vi "control tab sliding.vi"(10 "close(T)/open(F)":bool, 11 "String":string) -> ()   [LabVIEW 2017]
doc: "SciScan 1.2 160622"
uses:
  GFG/GFGfpRefGet.vi
  GFG/GFGnumericGet.vi
  GFG/GFG library.lvlib
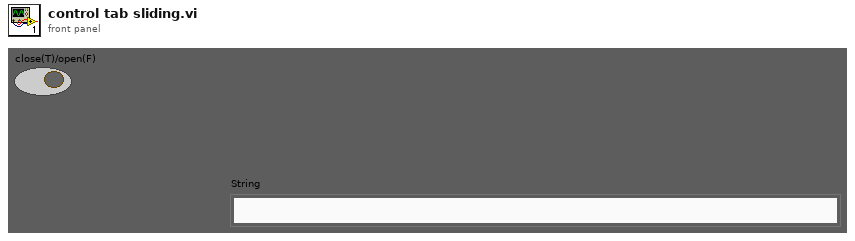
[diagram p1: front panel]
types:
  T1 = cluster{"WaveformChartRef":refnum<vi>, "DigitalRef":refnum<vi>, "ArrayRef":refnum<vi>, "TabControlRef":refnum<vi>, "EnumRef":refnum<vi>, "RingRef":refnum<vi>, "BooleanRef":refnum<vi>, "KnobRef":refnum<vi>, "SlideRef":refnum<vi>, "PathRef":refnum<vi>, "StringRef":refnum<vi>, "ComboBox":refnum<vi>, "WaveformGraphRef":refnum<vi>}
  T2 = cluster{"[0]":dbl, "[1]":dbl, "[2]":dbl, "[3]":dbl, "[4]":dbl, "[5]":dbl, "[6]":dbl, "[7]":dbl, "[8]":dbl}
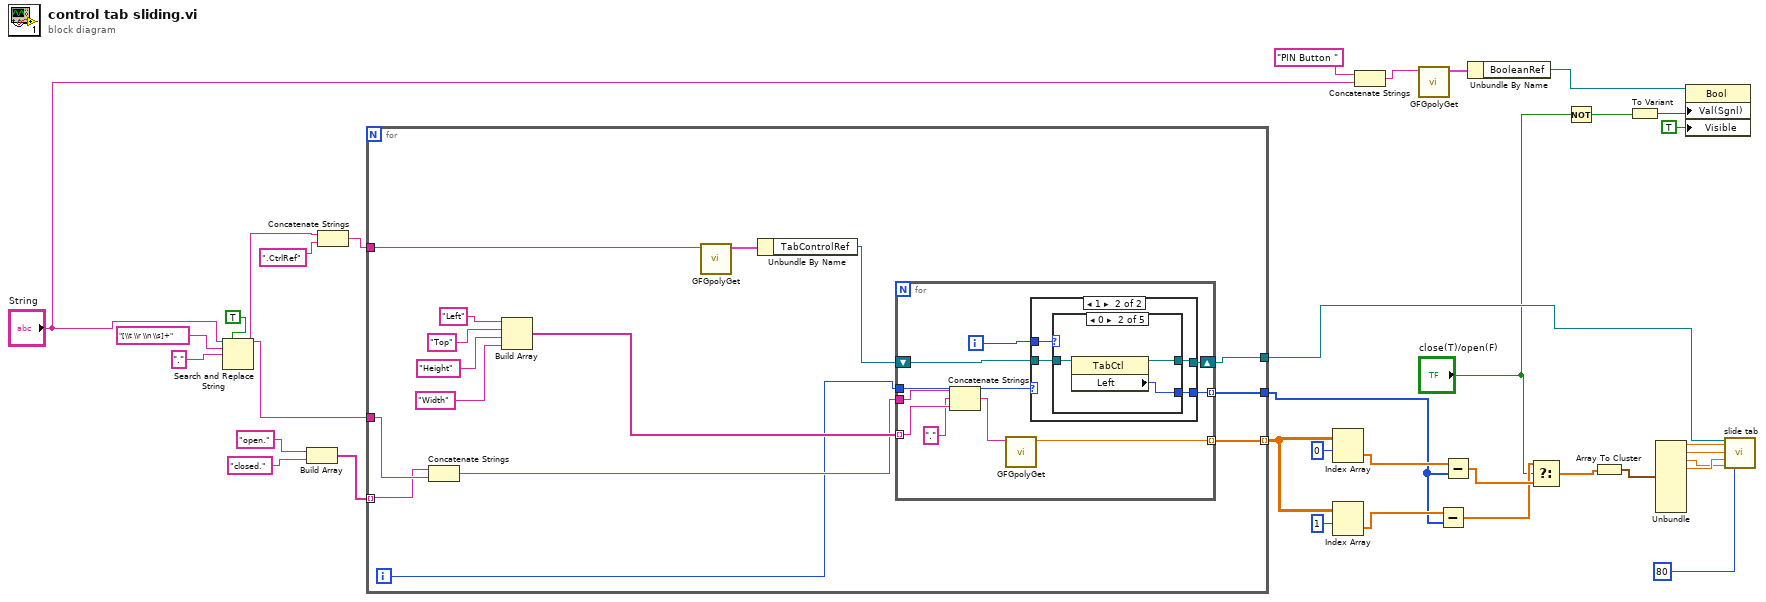
[diagram p0: block diagram]
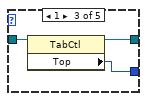
[diagram p4: hidden frame]
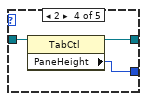
[diagram p5: hidden frame]
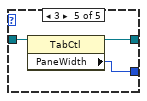
[diagram p6: hidden frame]
diagram:
  n1 = Search and Replace String(replace all?=TRUE ("replace all? (F)"), input string="String", search string="[\\t \\r \\n \\s]+", replace string="." ("replace string (\"\")")) -> (result string=w19:string)  [unwired: 4 in, 3 out]
  n2 = Build Array("open." ("String"), "closed." ("String")) -> (w29:string[])
  n3 = Concatenate Strings(w19, ".CtrlRef" ("search string")) -> (w17:string)
  n4 = for {
    tunnel: w19 -> [w47]
    tunnel: w29 -> [w46] mode=indexing
    tunnel: w17 -> [w35]
    tunnel: [w38] -> w23
    tunnel: [w37] -> w28 mode=indexing
    tunnel: [w36] -> w20
    i -> [w39]
    n5 = Concatenate Strings(w46, w47) -> (w40:string)
    n6 = Build Array("Left" ("replace string (\"\")"), "Top" ("replace string (\"\")"), "Height" ("replace string (\"\")"), "Width" ("replace string (\"\")")) -> (w41:string[])
    n7 = call-poly "GFGpolyGet.vi"("Variable Name in"=w35) -> ("output cluster"=w49:T1)  [unwired: 9 in, 1 out]
    n8 = Unbundle By Name(w49) -> ("TabControlRef"=w48:refnum<vi>)
    n9 = for {
      shift-right: [w57] -> w36
      shift-left: w48 -> [w58]
      tunnel: w40 -> [w51]
      tunnel: w41 -> [w55] mode=indexing
      tunnel: [w54] -> w37 mode=indexing
      tunnel: [w53] -> w38 mode=indexing
      tunnel: w39 -> [w52]
      i -> [w59]
      n10 = Concatenate Strings(w51, "." ("string"), w55) -> (w56:string)
      n11 = call-poly "GFGpolyGet.vi"("Variable Name in"=w56) -> ("Numeric"=w54:dbl)  [unwired: 8 in, 2 out]
      n12 = case shown="1" w52 {
        tunnel: w59 -> [_ w64]
        tunnel: w58 -> [w60 w63]
        tunnel: [w60 w62] -> w57
        tunnel: [_ w61] -> w53
        frame 0, Default {
        }
        frame 1 {
          n13 = case shown="0" w64 {
            tunnel: w63 -> [w65 w68 w71 w74 w77]
            tunnel: [w65 w67 w70 w73 w76] -> w62
            tunnel: [_ w66 w69 w72 w75] -> w61
            frame -1, Default {
            }
            frame 0 {
              n14 = property class="TabCtl"(reference=w68) -> (reference out=w67:refnum<vi>, "Left"=w66:i32)  [unwired: 1 in, 1 out]
            }
            frame 1 {
              n15 = property class="TabCtl"(reference=w71) -> (reference out=w70:refnum<vi>, "Top"=w69:i32)  [unwired: 1 in, 1 out]
            }
            frame 2 {
              n16 = property class="TabCtl"(reference=w74) -> (reference out=w73:refnum<vi>, "PaneHeight"=w72:u32)  [unwired: 1 in, 1 out]
            }
            frame 3 {
              n17 = property class="TabCtl"(reference=w77) -> (reference out=w76:refnum<vi>, "PaneWidth"=w75:u32)  [unwired: 1 in, 1 out]
            }
          }
        }
      }
    }
  }
  n18 = Index Array(array=w28, index (row)=0) -> (element=w27:dbl[])  [unwired: 1 in]
  n19 = Index Array(array=w28, index (row)=1) -> (element=w24:dbl[])  [unwired: 1 in]
  n20 = Concatenate Strings("PIN Button " ("string"), "String") -> (w3:string)
  n21 = call-poly "GFGpolyGet.vi"("Variable Name in"=w3) -> ("output cluster"=w4:T1)  [unwired: 9 in, 1 out]
  n22 = Subtract(x=w24, y=w23) -> (x-y=w13:dbl[])
  n23 = Subtract(x=w27, y=w23) -> (x-y=w14:dbl[])
  n24 = Unbundle By Name(w4) -> ("BooleanRef"=w5:refnum<vi>)
  n25 = Select(t=w13, s="close(T)/open(F)", f=w14) -> (s? t:f=w26:dbl[])
  n26 = Not(x="close(T)/open(F)") -> (.not. x?=w1:bool)
  n27 = Array To Cluster(array=w26) -> (cluster=w25:T2)
  n28 = To Variant(anything=w1) -> (Variant=w6:variant)
  n29 = Unbundle(w25) -> ("[0]"=w22:dbl, "[1]"=w21:dbl, "[2]"=w11:dbl, "[3]"=w12:dbl)  [unwired: 5 out]
  n30 = property class="Bool"(reference=w5, "Val(Sgnl)"=w6, "Visible"=TRUE) -> ()  [unwired: 1 in, 2 out]
  n31 = call "slide tab.vi"("Tab Ref In"=w20, "slide (right)"=w22, "slide (down)"=w21, "enlarge (width)"=w12, "enlarge (height)"=w11, "pixel shift"=80) -> ()  [unwired: 10 in]
